vi "Dispaly Error Window.vi"(4 "Deactive Save Error?":bool=TRUE, 6 "Delete Call Chain?":bool, 8 "error in (no error)":errorcluster, 9 "Event Source":T1, 10 "Custom Error":T2) -> (0 "error out":errorcluster)   [LabVIEW 2019, in "Error.lvclass"]
uses:
  Error.lvclass
  TypeDef/Custom Error List.ctl
  SubModules/LogsAbstract/TypeDef/Event Source.ctl
  SubModules/LogsAbstract/LogsAbstract.lvclass
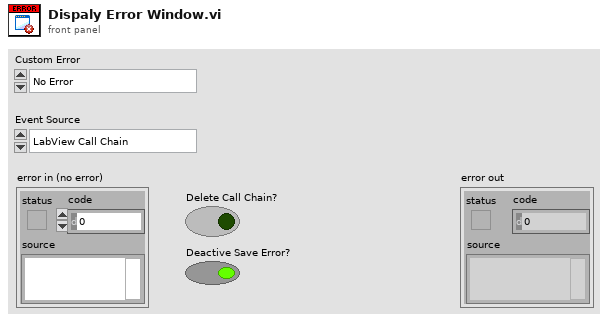
[diagram p1: front panel]
types:
  T1 = typedef "LogsAbstract.lvlib/LogsAbstract.lvclass/Event Source.ctl" = enum16{"LabView Call Chain", "Unknown", "< --- Modules --- >", "Core", "< --- SubModules --- >", "EventLog -> Core", "ErrorLog -> Core"}
  T2 = typedef "Error.lvclass/Custom Error List.ctl" = enum16{"No Error", "< --- System Errors --- >", "Lounching Modules Error", "StartApp Event Error", "Event Logging Error", "Modules Response Error", "< --- Process Errors --- >", "< --- Warnings --- >"}
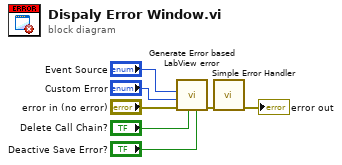
[diagram p0: block diagram]
diagram:
  n1 = call "Generate Error based LabView error.vi"("Deactive Save Error?"="Deactive Save Error?", "Delete Call Chain?"="Delete Call Chain?", "Error In"="error in (no error)", "Custom Error"="Custom Error", "Source"="Event Source") -> ("Error Out"=w5:errorcluster)  [unwired: 5 in, 1 out]
  n2 = call <vilib>:"Simple Error Handler.vi"("error in (no error)"=w5) -> ("error out"=→"error out":errorcluster)  [unwired: 4 in, 4 out]
